vi "WaveGraph Cursor(XY).vi"(8 "エラー入力（エラーなし）":errorcluster, 9 "色":u32(colorbox), 10 "名称":string, 11 "XYグラフref":refnum<vi>) -> (0 "エラー出力":errorcluster)   [LabVIEW 2014]
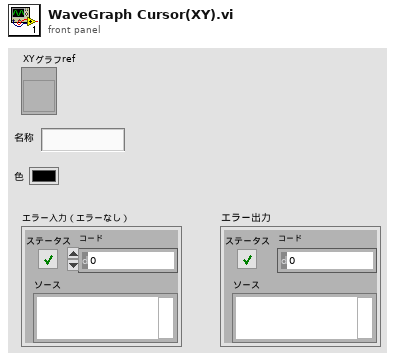
[diagram p1: front panel]
types:
  T1 = cluster{"Name":string, "Color":u32, "Style":u8, "Point Style":u8, "Name Visible":bool, "Allow Drag":bool, "Cursor Mode":u32, "Plot":i32, "Index":i32, "Position":cluster{"X":dbl, "Y":dbl}, "X Scale":u32, "Y Scale":u32, "Watch Plots":i32[], "Watch All Plots":bool, "Plot Area":i32, "Label Offset":cluster{"X":dbl, "Y":dbl}}
  T2 = typedef "LVCursorListTypeDef.ctl" = cluster{"Name":string, "Color":u32, "Style":u8, "Point Style":u8, "Name Visible":bool, "Allow Drag":bool, "Cursor Mode":u32, "Plot":i32, "Index":i32, "Position":cluster{"X":dbl, "Y":dbl}, "X Scale":u32, "Y Scale":u32, "Watch Plots":i32[], "Watch All Plots":bool, "Plot Area":i32, "Label Offset":cluster{"X":dbl, "Y":dbl}}[]
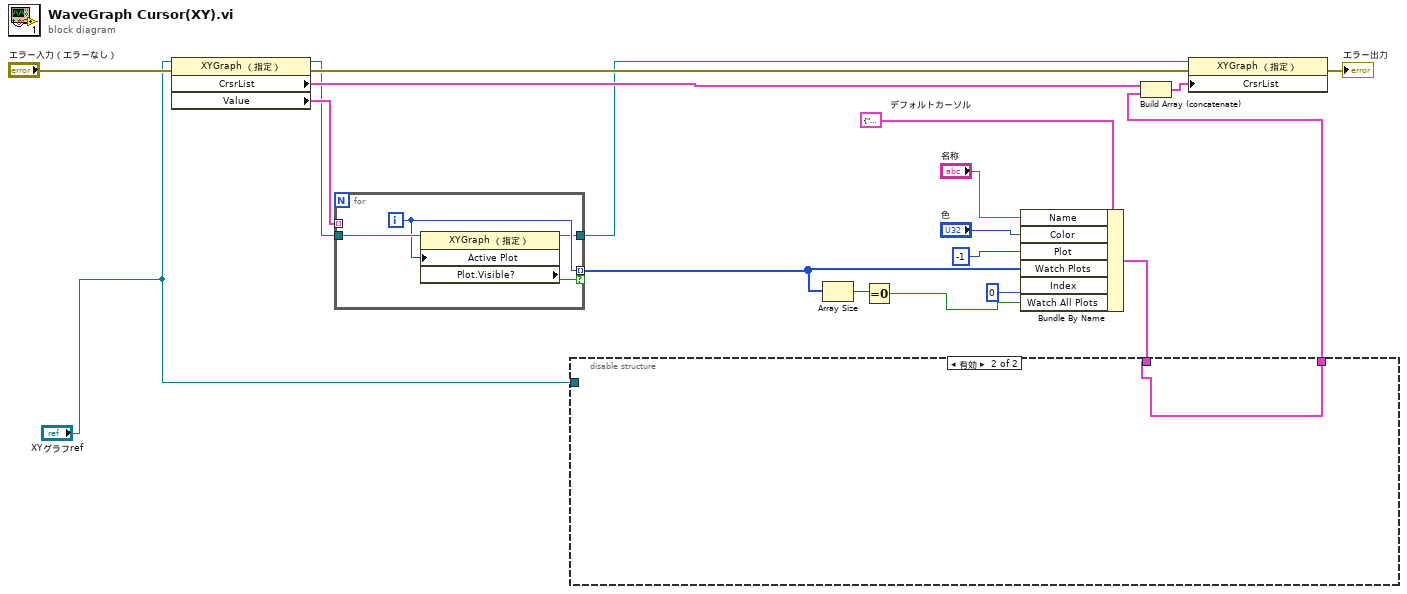
[diagram p0: block diagram]
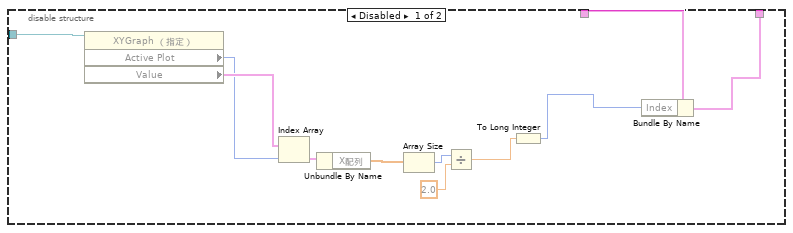
[diagram p2: hidden frame]
diagram:
  w10 = T1 {"Name"="カーソル0", "Color"=16776960, "Style"=2, "Point Style"=13, "Name Visible"=FALSE, "Allow Drag"=TRUE, "Cursor Mode"=2, "Plot"=-1, "Index"=42, "Position"={"X"=0.42, "Y"=43.0}, "X Scale"=0, "Y Scale"=0, "Watch Plots"=[], "Watch All Plots"=TRUE, "Plot Area"=0, "Label Offset"={"X"=-0.0012080536912751905, "Y"=172.10516252390056}}  # デフォルトカーソル
  n1 = property class="XYGraph （指定）"(reference="XYグラフref", error in="エラー入力（エラーなし）") -> (reference out=w5:refnum<vi>, error out=w12:errorcluster, "CrsrList"=w18:T2, "Value"=w17:cluster{"X配列":dbl[], "Y配列":dbl[]}[])
  n2 = for {
    tunnel: w5 -> [w23]
    tunnel: w17 -> [_] mode=indexing
    tunnel: [w22] -> w4 mode=indexing if=w21
    tunnel: [w20] -> w6
    i -> [w22]
    n3 = property class="XYGraph （指定）"(reference=w23, "Active Plot"=w22) -> (reference out=w20:refnum<vi>, "Plot.Visible?"=w21:bool)  [unwired: 1 in, 1 out]
  }
  n4 = Array Size(array=w4) -> (size(s)=w3:i32)
  n5 = Equal To 0?(x=w3) -> (x = 0?=w2:bool)
  n6 = Bundle By Name(cluster=w10, "Name"="名称", "Color"="色", "Plot"=-1, "Watch Plots"=w4, "Index"=0, "Watch All Plots"=w2) -> (w8:T1)
  n7 = disable-structure shown="有効" {
    disable-tunnel: w8 -> [w34 w35]
    disable-tunnel: [w33 w35] -> w7
    disable-tunnel: "XYグラフref" -> [w32 _]
    frame Disabled {
      n8 = property class="XYGraph （指定）"(reference=w32) -> ("Active Plot"=w30:u32, "Value"=w31:cluster{"X配列":dbl[], "Y配列":dbl[]}[])  [unwired: 1 in, 2 out]
      n9 = Index Array(array=w31, index=w30) -> (element=w28:cluster{"X配列":dbl[], "Y配列":dbl[]})
      n10 = Unbundle By Name(w28) -> ("X配列"=w27:dbl[])
      n11 = Array Size(array=w27) -> (size(s)=w26:i32)
      n12 = Divide(x=w26, y=2.0) -> (x/y=w24:dbl)
      n13 = To Long Integer(number=w24) -> (32bit integer=w29:i32)
      n14 = Bundle By Name(cluster=w34, "Index"=w29) -> (w33:T1)
    }
    frame Enabled {
    }
  }
  n15 = Build Array (concatenate)(w18, w7) -> (w14:T2)
  n16 = property class="XYGraph （指定）"(reference=w6, error in=w12, "CrsrList"=w14) -> (error out=→"エラー出力":errorcluster)  [unwired: 1 out]
